vi "Do.vi"(8 "error in (no error)":errorcluster, 10 "Actor in":refnum<class "Actor.lvclass">, 11 "Visualize FFT Msg":refnum<class "Visualize FFT Msg.lvclass">) -> (0 "error out":errorcluster, 2 "Actor out":refnum<class "Actor.lvclass">)   [LabVIEW 2025, in "Application Manager.lvlib" / "Visualize FFT Msg.lvclass"]
doc: "This VI delivers the message to the actor by calling the appropriate method(s) on the actor."
uses:
  Visualize FFT Msg.lvclass
  Visualize FFT Msg.lvclass/Visualize FFT Msg.ctl
  36aa740b-de47-447a-9ae4-3731dfe514ec.vi
  Application Manager/Application Manager.lvclass
  <vilib>/ActorFramework/Actor/Actor.lvclass
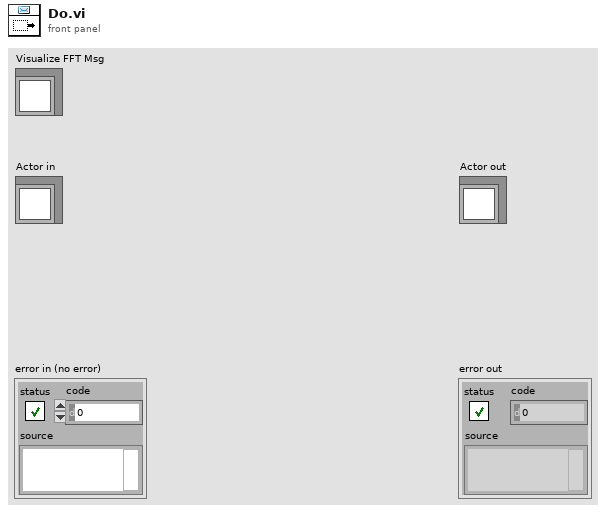
[diagram p1: front panel]
types:
  T1 = typedef "UI Root.lvlib/UI Root.lvclass/FFT Plot Data.ctl" = cluster{"FFT":refnum<data-value>, "df":dbl, "d0":dbl}
  T2 = typedef "UI Root.lvlib/UI Root.lvclass/Signal Density Plot Data.ctl" = cluster{"Plot":refnum<data-value>, "Plot Scale":cluster{"X Scale":T3, "Y Scale":T3}}
  T3 = typedef "LVOffsetAndMultiplierTypeDef.ctl" = cluster{"Offset":dbl, "Multiplier":dbl}
  T4 = typedef "UI Root.lvlib/UI Root.lvclass/Frequency Metadata.ctl" = cluster{"df":dbl, "d0":dbl}
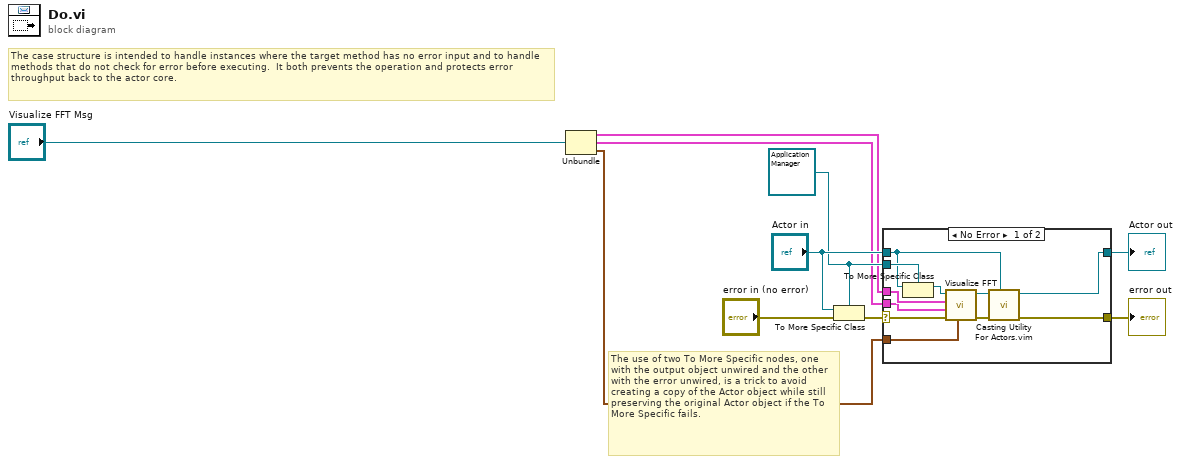
[diagram p0: block diagram]
diagram:
  w5 = refnum<class "Application Manager.lvclass"> refnum ("Actor in")
  # "The use of two To More Specific nodes, one with the output object unwired and the other with the error unwired, is a trick to avoid creating a copy of the Actor object while still preserving the original Actor object if the To More Specific fails."
  # "The case structure is intended to handle instances where the target method has no error input and to handle methods that do not check for error before executing.  It both prevents the operation and protects error throughput back to the actor core."
  n1 = Unbundle("Visualize FFT Msg") -> (w3:T1, w2:T2, w1:T4)
  n2 = To More Specific Class(target class=w5, reference="Actor in", error in="error in (no error)") -> (error out=w4:errorcluster)  [unwired: 1 out]
  n3 = case shown="No Error" w4 {
    selector: w4 -> [w21 w23]
    tunnel: [w15 w23] -> w10
    tunnel: [w16 w22] -> w9
    tunnel: "Actor in" -> [w18 w22]
    tunnel: w5 -> [w19 _]
    tunnel: w3 -> [w13 _]
    tunnel: w2 -> [w12 _]
    tunnel: w1 -> [w11 _]
    frame No Error {
      n4 = To More Specific Class(target class=w19, reference=w18) -> (specific class reference=w20:refnum<class "Application Manager.lvclass">)  [unwired: 1 in, 1 out]
      n5 = call-dynamic "Visualize FFT.vi"("Frequency Metedata"=w11, "error in (no error)"=w21, "Signal Density Plot"=w12, "FFT Data"=w13, "Application Manager in"=w20) -> ("error out"=w14:errorcluster, "Application Manager out"=w17:refnum<class "Application Manager.lvclass">)  [unwired: 5 in]
      n6 = call "Casting Utility For Actors.vim"("type"=w18, "error in (no error)"=w14, "Actor in"=w17) -> ("error out"=w15:errorcluster, "Actor out"=w16:refnum<class "Actor.lvclass">)  [unwired: 7 in]
    }
    frame Error {
      # "If type check fails, pass the original object out again."
    }
  }
  "error out" <- w10
  "Actor out" <- w9
